vi "TransferItems.vi"(8 "error in":errorcluster, 10 "Session":refnum<class "Session.lvclass">, 11 "TransferFiles in":refnum<class "TransferFiles-Get.lvclass">) -> (0 "error out":errorcluster, 3 "FileTransfer out":refnum<class "TransferFiles-Get.lvclass">)   [LabVIEW 2015, in "WinSCP.lvlib" / "TransferFiles-Get.lvclass"]
uses:
  TransferFiles-Get.lvclass
  Session/Session.lvclass
  C:/Program Files (x86)/WinSCP/WinSCPnet.dll
  Program Files (x86)/WinSCP/WinSCPnet.dll
  FileTransferOptions/FileTransferOptions.lvclass
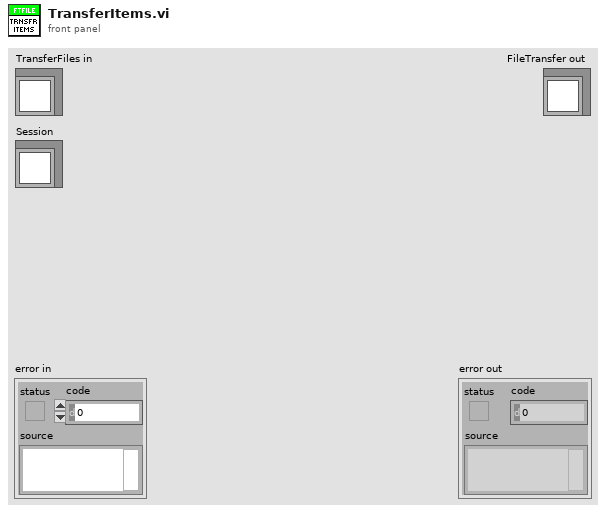
[diagram p1: front panel]
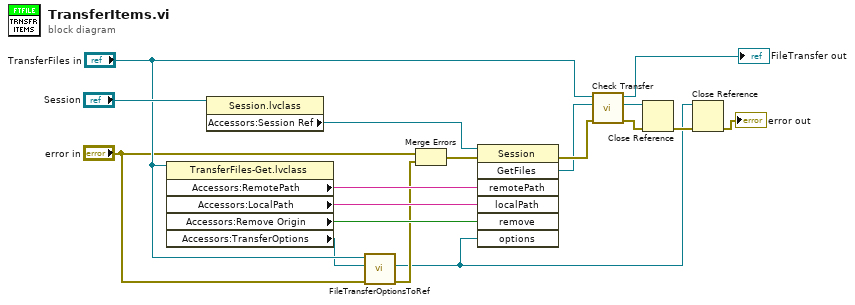
[diagram p0: block diagram]
diagram:
  n1 = property class="TransferFiles-Get.lvclass"(reference="TransferFiles in") -> ("Accessors:RemotePath"=w17:string, "Accessors:LocalPath"=w16:string, "Accessors:Remove Origin"=w15:bool, "Accessors:TransferOptions"=w7:refnum<class "FileTransferOptions.lvclass">)  [unwired: 1 in, 2 out]
  n2 = property class="Session.lvclass"(reference="Session") -> ("Accessors:Session Ref"=w11:refnum<k24>)  [unwired: 1 in, 2 out]
  n3 = call-dynamic "FileTransferOptionsToRef.vi"("error in (no error)"="error in", "FileTransferOptions"=w7, "FileTransfer in"="TransferFiles in") -> ("error out"=w4:errorcluster, "TransferOptions Ref"=w1:refnum<k24>)  [unwired: 7 in]
  n4 = Merge Errors("error in", w4) -> (w5:errorcluster)
  n5 = invoke class="Session" method="GetFiles"(reference=w11, error in=w5, "remotePath"=w17, "localPath"=w16, "remove"=w15, "options"=w1) -> (error out=w18:errorcluster, "GetFiles"=w13:refnum<k24>)  [unwired: 1 in, 5 out]
  n6 = call-dynamic "Check Transfer.vi"("error in"=w18, "TransferOperationResult in"=w13, "FileTransfer in"="TransferFiles in") -> ("error out"=w14:errorcluster, "TransferOperationResult out"=w10:refnum<k24>, "FileTransfer out"=→"FileTransfer out":refnum<class "TransferFiles-Get.lvclass">)  [unwired: 6 in]
  n7 = Close Reference(reference=w10, error in (no error)=w14) -> (error out=w3:errorcluster)
  n8 = Close Reference(reference=w1, error in (no error)=w3) -> (error out=→"error out":errorcluster)
